vi "rpm_meter.vi"() -> ()   [LabVIEW 2009]
uses:
  <vilib>/measure/matone.llb/Extract Single Tone Information N Chan.vi
  <vilib>/measure/NI_MAPro.lvlib
panel:
  out "GPM":dbl
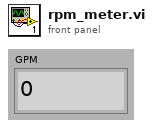
[diagram p1: front panel]
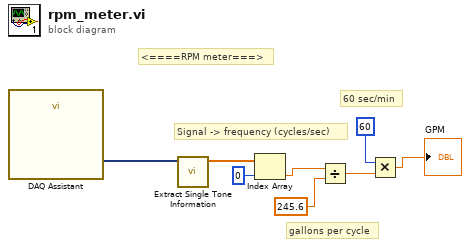
[diagram p0: block diagram]
diagram:
  # "<====RPM meter===>"
  # "60 sec/min"
  # "gallons per cycle"
  # "Signal -> frequency (cycles/sec)"
  n1 = call "DAQ Assistant"() -> ("data"=w8:dynamicdata)  [unwired: 17 in, 2 out]
  n2 = call-poly <vilib>:"Extract Single Tone Information.vi"("time signals in"=w8) -> ("detected frequencies"=w7:dbl[])  [unwired: 5 in, 5 out]
  n3 = Index Array(array=w7, index=0) -> (element=w5:dbl)
  n4 = Divide(x=w5, y=245.6) -> (x/y=w3:dbl)
  n5 = Multiply(x=60, y=w3) -> (x*y=→"GPM":dbl)
